vi "px2um.vi"(1 "px":sgl, 2 "Size factor":dbl, 3 "Field of view":dbl) -> (0 "um":dbl)   [LabVIEW 2015]
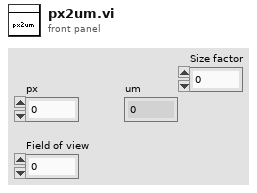
[diagram p1: front panel]
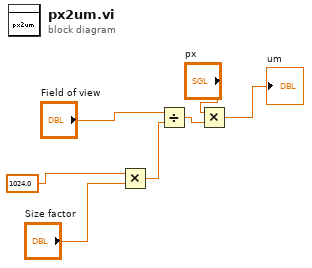
[diagram p0: block diagram]
diagram:
  n1 = Multiply(x=1024.0 ("y"), y="Size factor") -> (x*y=w1:dbl)
  n2 = Divide(x="Field of view", y=w1) -> (x/y=w6:dbl)
  n3 = Multiply(x="px", y=w6) -> (x*y=→"um":dbl)
